vi "Inc16.vi"(8 "a":bool[](array[boolean])=[FALSE, FALSE, FALSE, FALSE, FALSE, FALSE, FALSE, FALSE, FALSE, FALSE, FALSE, FALSE, FALSE, FALSE, FALSE, FALSE]) -> (2 "out":bool[](array[boolean]))   [LabVIEW 2014]
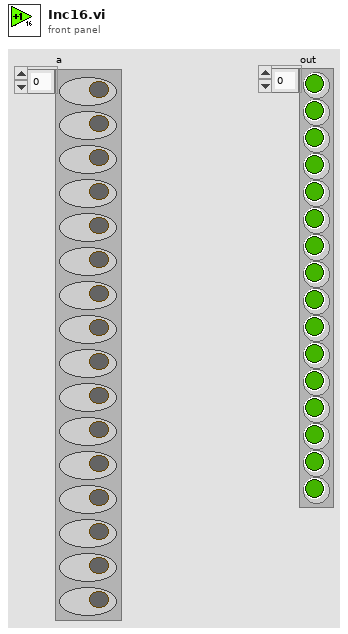
[diagram p1: front panel]
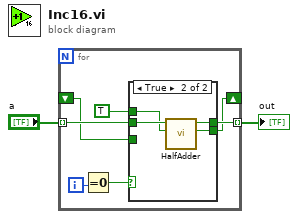
[diagram p0: block diagram]
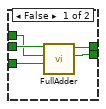
[diagram p2: hidden frame]
diagram:
  n1 = for {
    tunnel: "a" -> [w7] mode=indexing
    tunnel: [w6] -> w1 mode=indexing
    shift-right: [w5] -> _
    shift-left: _ -> [w4]
    i -> [w9]
    n2 = Equal To 0?(x=w9) -> (x = 0?=w8:bool)
    n3 = case shown="True" w8 {
      tunnel: w7 -> [w14 w18]
      tunnel: [w12 w17] -> w6
      tunnel: [w11 w16] -> w5
      tunnel: w4 -> [w13 _]
      tunnel: TRUE ("b") -> [w10 w15]
      frame False {
        n4 = call "FullAdder.vi"("c"=w13, "b"=w10, "a"=w14) -> ("carry"=w11:bool, "sum"=w12:bool)  [unwired: 7 in]
      }
      frame True {
        n5 = call "HalfAdder.vi"("b"=w15, "a"=w18) -> ("carry"=w16:bool, "sum"=w17:bool)  [unwired: 8 in]
      }
    }
  }
  "out" <- w1
